vi "getPubKey.vi"(0 "HGF_GPG.lvclass in":refnum<class "HGF_GPG.lvclass">, 5 "error in (no error)":errorcluster) -> (14 "HGF_GPG.lvclass out":refnum<class "HGF_GPG.lvclass">, 16 "public Key":string, 19 "error out":errorcluster)   [LabVIEW 2012, in "HGF_GPG.lvlib" / "HGF_GPG.lvclass"]
uses:
  HGF_GPG.lvclass
  HGF_GPG.lvclass/HGF_GPG.ctl
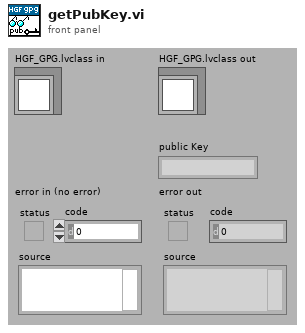
[diagram p1: front panel]
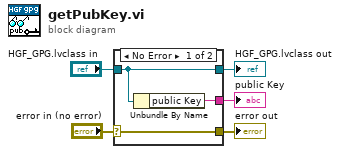
[diagram p0: block diagram]
diagram:
  n1 = case shown="No Error" "error in (no error)" {
    selector: "error in (no error)" -> [w8 w9]
    tunnel: [w8 w9] -> w4
    tunnel: [w7 w10] -> w2
    tunnel: "HGF_GPG.lvclass in" -> [w7 w10]
    tunnel: [w6 _] -> w1
    frame No Error {
      n2 = Unbundle By Name(w7) -> ("public Key"=w6:string)
    }
    frame Error {
    }
  }
  "error out" <- w4
  "HGF_GPG.lvclass out" <- w2
  "public Key" <- w1
